vi "Create Evaluation String.vi"(8 "error in (no error)":errorcluster, 10 "Evaluation String":string, 11 "Test in":refnum<class "Test.lvclass">) -> (0 "error out":errorcluster, 3 "Test out":refnum<class "Test.lvclass">)   [LabVIEW 2018, in "Test.lvclass"]
uses:
  Test.lvclass
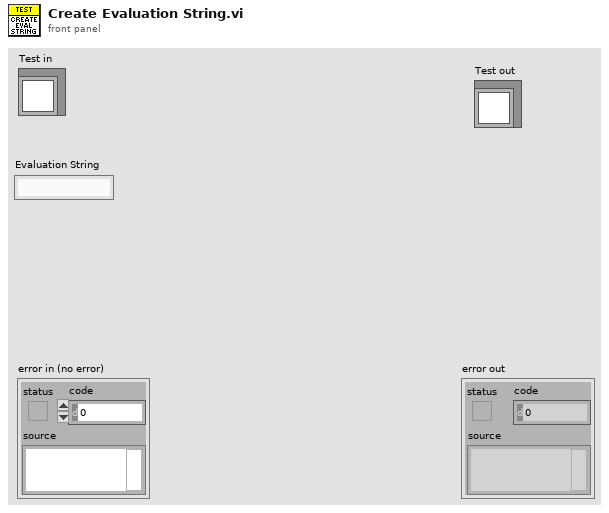
[diagram p1: front panel]
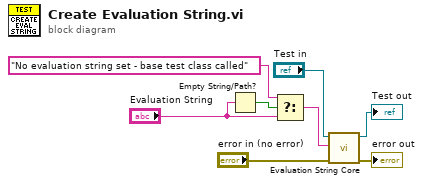
[diagram p0: block diagram]
diagram:
  n1 = Empty String/Path?(string/path="Evaluation String") -> (empty?=w4:bool)
  n2 = Select(t="No evaluation string set - base test class called", s=w4, f="Evaluation String") -> (s? t:f=w1:string)
  n3 = call "Evaluation String Core.vi"("error in (no error)"="error in (no error)", "Evaluation String"=w1, "Test in"="Test in") -> ("error out"=→"error out":errorcluster, "Test out"=→"Test out":refnum<class "Test.lvclass">)  [unwired: 7 in]
